vi "Air Flow Meters.vi"() -> ()   [LabVIEW 2017]
uses:
  Flow Set AFM.vi
  Flow Out AFM.vi
  Halt AFM.vi
  <vilib>/addons/control/pid/pid.llb/PID Control Input Filter (DBL).vi
  <vilib>/addons/control/pid/pid.llb/PID Advanced (DBL).vi
  <vilib>/addons/control/pid/NI_PID_pid.lvlib
panel:
  in  "Flowrate Setpoint":dbl=100.0 caption="(SCFM)" format="%.1f"
  in  "Set Manual Valve Position":dbl(slide)=100.0 scale=0.0..100.0
  out "Control Valve":dbl(slide) scale=0.0..100.0
  in  "Manual Control Override":bool
  in  "Td":dbl caption="(min)"
  in  "Ti":dbl=0.5 caption="(min)"
  in  "Kc":dbl=-0.33
  in  "Enable 3":bool
  out "Saving Data 3":bool
  out "Data Point Count":i32
  in  "Specify Time between Data Points (sec)":dbl=1.0
  in  "Cancel Data Collection":bool
  in  "Specify number of data points":i16=1
  out "Mass Flow Meter":dbl caption="SCFM" format="%.1f"
  out "Rotameter Entrance Pressure":dbl format="%.2f"
  out "Orifice Entrance Pressure":dbl format="%.2f"
  out "Orifice Delta P":dbl format="%.2f"
  out "Nozzle Entrance Pressure":dbl format="%.2f"
  out "Nozzle Delta P":dbl caption="\"WC" format="%.2f"
  out "Venturi Entrance Pressure":dbl format="%.2f"
  out "Venturi Delta P":dbl format="%.2f"
  out "Pitot Entrance Pressure":dbl format="%.2f"
  out "Pitot Delta P":dbl caption="\"WC" format="%.2f"
  in  "stop":bool
  out "Temperature 4":dbl format="%.1g"
  out "Temperature 3":dbl format="%.1g"
  out "Temperature 2":dbl format="%.1g"
  out "Temperature 1":dbl format="%.1g"
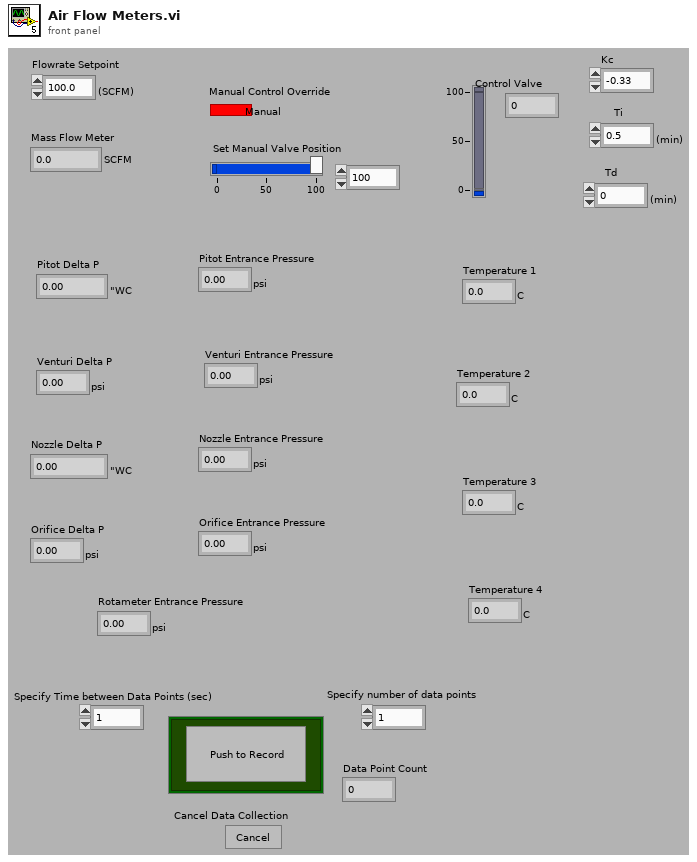
[diagram p1: front panel]
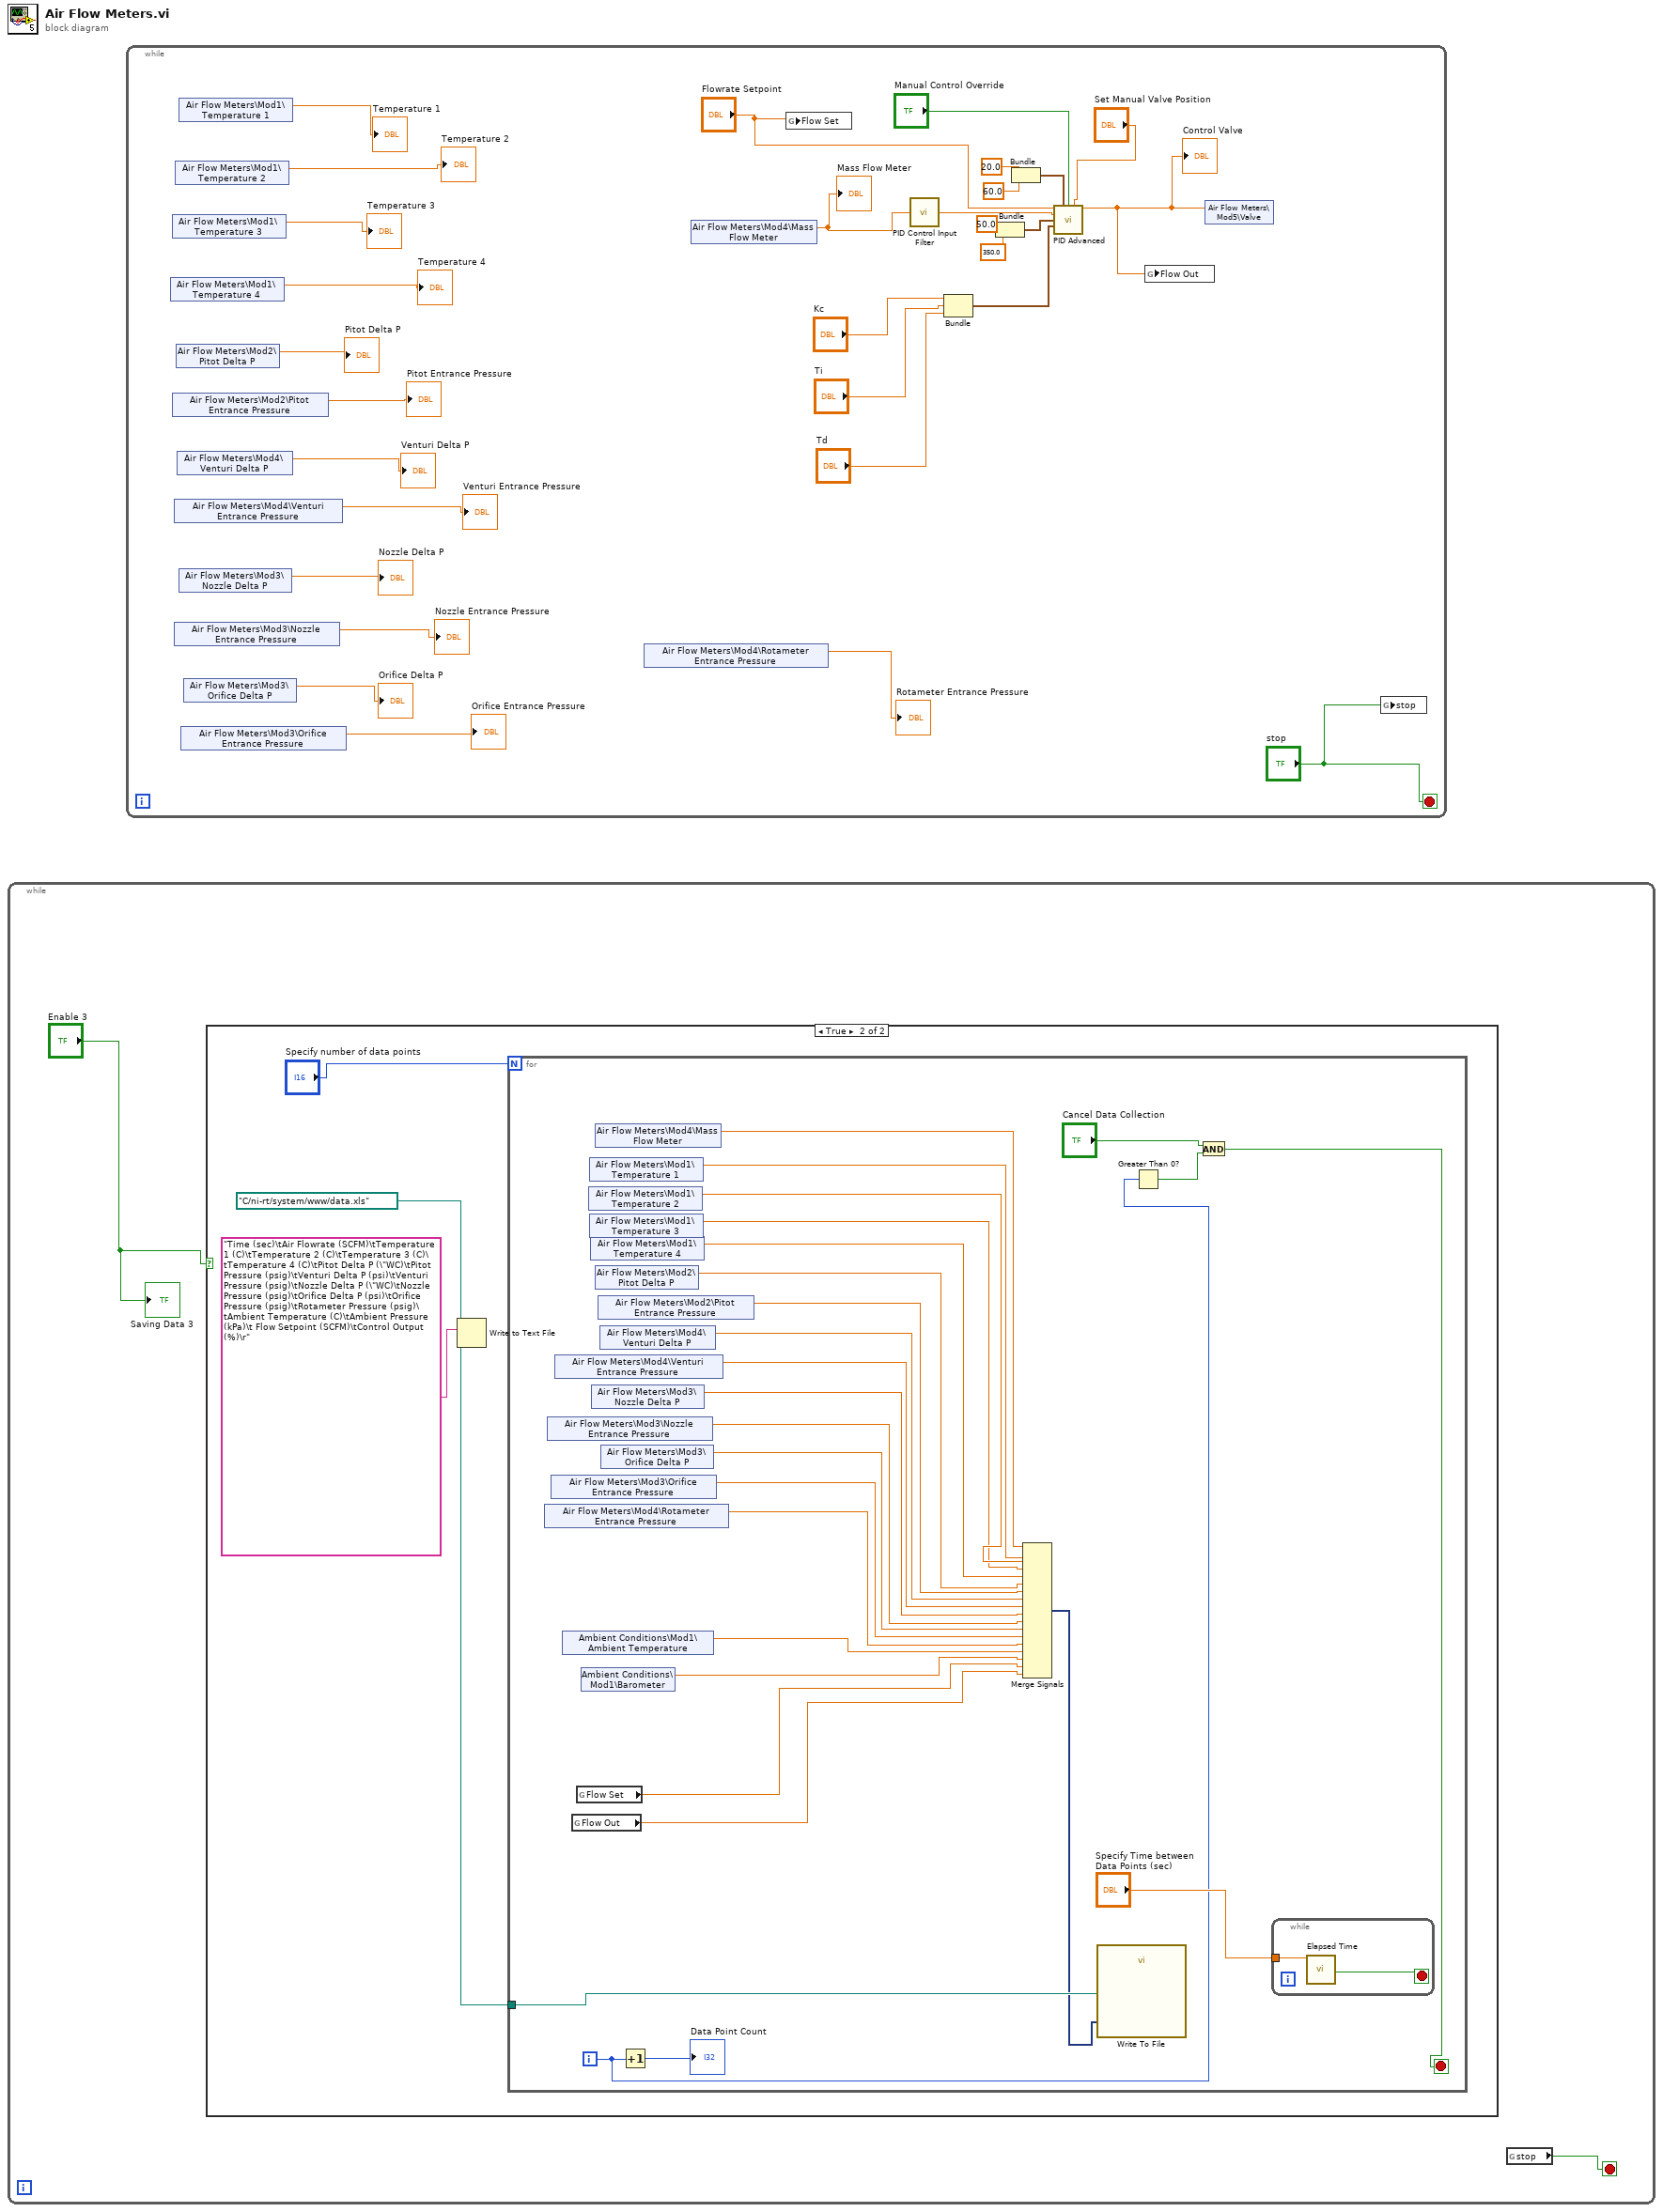
[diagram p0: block diagram]
diagram:
  n1 = while {
    stop <- w1 stop-if-true
    n2 = case shown="True" "Enable 3" {
      frame False {
      }
      frame True {
        w4 = path "C:/ni-rt/system/www/data.xls" ("Filename")
        n3 = Write to Text File(file (use dialog)=w4, text="Time (sec)\tAir Flowrate (SCFM)\tTemperature 1 (C)\tTemperature 2 (C)\tTemperature 3 (C)\tTemperature 4 (C)\tPitot Delta P (\"WC)\tPitot Pressure (psig)\tVenturi Delta P (psi)\tVenturi Pressure (psig)\tNozzle Delta P (\"WC)\tNozzle Pressure (psig)\tOrifice Delta P (psi)\tOrifice Pressure (psig)\tRotameter Pressure (psig)\tAmbient Temperature (C)\tAmbient Pressure (kPa)\t Flow Setpoint (SCFM)\tControl Output (%)\r") -> ()  [unwired: 2 in, 3 out]
        n4 = for {
          N: "Specify number of data points" -> [_]
          tunnel: w4 -> [w31]
          i -> [w25]
          stop <- w22 stop-if-true
          n5 = shared-variable "Air Flow Meters\\Mod4\\Rotameter Entrance Pressure"() -> (w10:dbl)  [unwired: 1 in, 1 out]
          n6 = shared-variable "Air Flow Meters\\Mod3\\Nozzle Entrance Pressure"() -> (w13:dbl)  [unwired: 1 in, 1 out]
          n7 = shared-variable "Air Flow Meters\\Mod3\\Orifice Entrance Pressure"() -> (w11:dbl)  [unwired: 1 in, 1 out]
          n8 = shared-variable "Air Flow Meters\\Mod4\\Venturi Entrance Pressure"() -> (w15:dbl)  [unwired: 1 in, 1 out]
          n9 = shared-variable "Ambient Conditions\\Mod1\\Ambient Temperature"() -> (w9:dbl)  [unwired: 1 in, 1 out]
          n10 = global read "Flow Out AFM.vi" "Flow Out"() -> (w6:dbl)
          n11 = global read "Flow Set AFM.vi" "Flow Set"() -> (w7:dbl)
          n12 = shared-variable "Ambient Conditions\\Mod1\\Barometer"() -> (w8:dbl)  [unwired: 1 in, 1 out]
          n13 = shared-variable "Air Flow Meters\\Mod1\\Temperature 2"() -> (w28:dbl)  [unwired: 1 in, 1 out]
          n14 = shared-variable "Air Flow Meters\\Mod1\\Temperature 1"() -> (w29:dbl)  [unwired: 1 in, 1 out]
          n15 = shared-variable "Air Flow Meters\\Mod1\\Temperature 3"() -> (w21:dbl)  [unwired: 1 in, 1 out]
          n16 = shared-variable "Air Flow Meters\\Mod1\\Temperature 4"() -> (w20:dbl)  [unwired: 1 in, 1 out]
          n17 = shared-variable "Air Flow Meters\\Mod3\\Nozzle Delta P"() -> (w14:dbl)  [unwired: 1 in, 1 out]
          n18 = shared-variable "Air Flow Meters\\Mod4\\Mass Flow Meter"() -> (w17:dbl)  [unwired: 1 in, 1 out]
          n19 = shared-variable "Air Flow Meters\\Mod2\\Pitot Delta P"() -> (w19:dbl)  [unwired: 1 in, 1 out]
          n20 = shared-variable "Air Flow Meters\\Mod2\\Pitot Entrance Pressure"() -> (w18:dbl)  [unwired: 1 in, 1 out]
          n21 = shared-variable "Air Flow Meters\\Mod4\\Venturi Delta P"() -> (w16:dbl)  [unwired: 1 in, 1 out]
          n22 = shared-variable "Air Flow Meters\\Mod3\\Orifice Delta P"() -> (w12:dbl)  [unwired: 1 in, 1 out]
          n23 = Increment(x=w25) -> (x+1=→"Data Point Count":i32)
          n24 = Merge Signals(w17, w29, w28, w21, w20, w19, w18, w16, w15, w14, w13, w12, w11, w10, w9, w8, w7, w6) -> (w27:dynamicdata)
          n25 = call "Write To File"("Signals"=w27, "Filename"=w31) -> ()  [unwired: 15 in, 3 out]
          n26 = Greater Than 0?(x=w25) -> (x > 0?=w23:bool)
          n27 = And(x="Cancel Data Collection", y=w23) -> (x .and. y?=w22:bool)
          n28 = while {
            tunnel: "Specify Time between Data Points (sec)" -> [w32]
            stop <- w33 stop-if-true
            n29 = call "Elapsed Time"("Time Target (s)"=w32) -> ("Time has Elapsed"=w33:bool)  [unwired: 11 in, 7 out]
          }
        }
      }
    }
    n30 = global read "Halt AFM.vi" "stop"() -> (w1:bool)
    "Saving Data 3" <- "Enable 3"
  }
  n31 = while {
    stop <- "stop" stop-if-true
    n32 = shared-variable "Air Flow Meters\\Mod1\\Temperature 4"() -> (→"Temperature 4":dbl)  [unwired: 1 in, 1 out]
    n33 = shared-variable "Air Flow Meters\\Mod1\\Temperature 3"() -> (→"Temperature 3":dbl)  [unwired: 1 in, 1 out]
    n34 = shared-variable "Air Flow Meters\\Mod2\\Pitot Entrance Pressure"() -> (→"Pitot Entrance Pressure":dbl)  [unwired: 1 in, 1 out]
    n35 = shared-variable "Air Flow Meters\\Mod4\\Venturi Entrance Pressure"() -> (→"Venturi Entrance Pressure":dbl)  [unwired: 1 in, 1 out]
    n36 = shared-variable "Air Flow Meters\\Mod3\\Nozzle Entrance Pressure"() -> (→"Nozzle Entrance Pressure":dbl)  [unwired: 1 in, 1 out]
    n37 = shared-variable "Air Flow Meters\\Mod1\\Temperature 2"() -> (→"Temperature 2":dbl)  [unwired: 1 in, 1 out]
    n38 = shared-variable "Air Flow Meters\\Mod2\\Pitot Delta P"() -> (→"Pitot Delta P":dbl)  [unwired: 1 in, 1 out]
    n39 = shared-variable "Air Flow Meters\\Mod4\\Venturi Delta P"() -> (→"Venturi Delta P":dbl)  [unwired: 1 in, 1 out]
    n40 = shared-variable "Air Flow Meters\\Mod1\\Temperature 1"() -> (→"Temperature 1":dbl)  [unwired: 1 in, 1 out]
    n41 = shared-variable "Air Flow Meters\\Mod3\\Nozzle Delta P"() -> (→"Nozzle Delta P":dbl)  [unwired: 1 in, 1 out]
    n42 = shared-variable "Air Flow Meters\\Mod3\\Orifice Entrance Pressure"() -> (→"Orifice Entrance Pressure":dbl)  [unwired: 1 in, 1 out]
    n43 = shared-variable "Air Flow Meters\\Mod3\\Orifice Delta P"() -> (→"Orifice Delta P":dbl)  [unwired: 1 in, 1 out]
    n44 = shared-variable "Air Flow Meters\\Mod4\\Rotameter Entrance Pressure"() -> (→"Rotameter Entrance Pressure":dbl)  [unwired: 1 in, 1 out]
    n45 = shared-variable "Air Flow Meters\\Mod4\\Mass Flow Meter"() -> (w34:dbl)  [unwired: 1 in, 1 out]
    "Mass Flow Meter" <- w34
    n46 = global write "Flow Set AFM.vi" "Flow Set"("Flowrate Setpoint") -> ()
    n47 = call-poly <vilib>:"PID Control Input Filter.vi"("input"=w34) -> ("output"=w35:dbl)  [unwired: 4 in]
    n48 = Bundle("Kc"="Kc", "Ti"="Ti", "Td"="Td") -> (w46:cluster{"Kc":dbl, "Ti":dbl, "Td":dbl})  [unwired: 1 in]
    n49 = Bundle(50.0, 350.0) -> (w40:cluster{dbl, dbl})  [unwired: 1 in]
    n50 = Bundle(20.0, 60.0) -> (w49:cluster{dbl, dbl})  [unwired: 1 in]
    n51 = call-poly <vilib>:"PID Advanced.vi"("setpoint"="Flowrate Setpoint", "output range"=w49, "auto? (T)"="Manual Control Override", "manual control"="Set Manual Valve Position", "process variable"=w35, "setpoint range"=w40, "PID gains"=w46) -> ("output"=w38:dbl)  [unwired: 7 in, 1 out]
    "Control Valve" <- w38
    n52 = global write "Flow Out AFM.vi" "Flow Out"(w38) -> ()
    n53 = shared-variable "Air Flow Meters\\Mod5\\Valve"(w38) -> ()  [unwired: 1 in, 1 out]
    n54 = global write "Halt AFM.vi" "stop"("stop") -> ()
  }
